vi "Init NetCPU.vi"(6 "instVIref":T1, 9 "target location":string, 11 "NetCPU in":refnum<class "NetCPU.lvclass">) -> (3 "NetCPU out":refnum<class "NetCPU.lvclass">)   [LabVIEW 2020, in "NI_TargetHelper.lvlib" / "NetCPU.lvclass"]
uses:
  <vilib>/TargetSupport/NI_TargetHelper/NetCPU/NetCPU.lvclass
  <vilib>/TargetSupport/NI_TargetHelper/Instance VIref.ctl
  <vilib>/TargetSupport/NI_TargetHelper/NetCPU/NetCPU.lvclass/NetCPU.ctl
  <vilib>/TargetSupport/NI_TargetHelper/NI_TargetHelper.lvlib
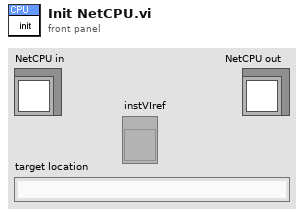
[diagram p1: front panel]
types:
  T1 = typedef "NI_TargetHelper.lvlib/Instance VIref.ctl" = refnum<vi>
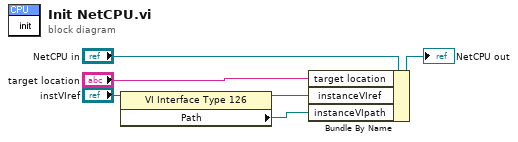
[diagram p0: block diagram]
diagram:
  n1 = property class="VI Interface Type 126"(reference="instVIref") -> (reference out=w2:T1, "Path"=w1:path)  [unwired: 1 in, 1 out]
  n2 = Bundle By Name(cluster="NetCPU in", "target location"="target location", "instanceVIref"=w2, "instanceVIpath"=w1) -> (→"NetCPU out":refnum<class "NetCPU.lvclass">)
